vi "RobotStatus.vi"(0 "Universal Robot.lvclass in":refnum<class "Universal Robot.lvclass">, 5 "error in (no error)":errorcluster) -> (14 "Universal Robot.lvclass out":refnum<class "Universal Robot.lvclass">, 15 "Robot Status":T1, 19 "error out":errorcluster)   [LabVIEW 2019, in "Universal Robot.lvclass"]
uses:
  Universal Robot.lvclass
  RobotStatus.ctl
  RobotMode.ctl
  OperationalMode.ctl
  SafetyStatus.ctl
  Universal Robot.lvclass/Universal Robot.ctl
  Client Interfaces/Dashboard Server/Dashboard Server.lvclass
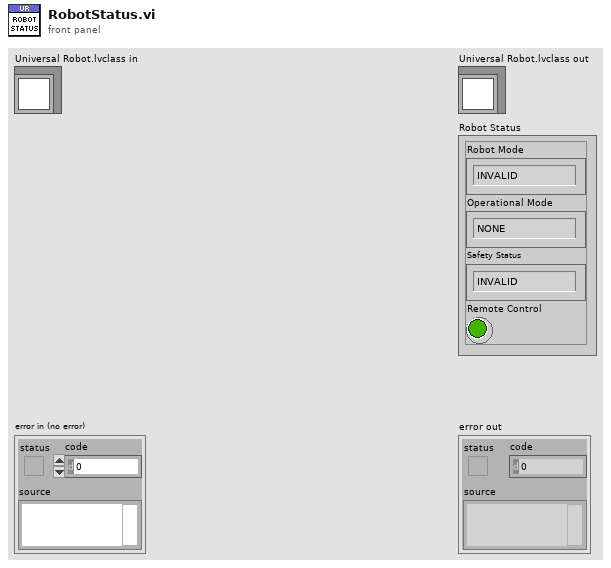
[diagram p1: front panel]
types:
  T1 = typedef "Universal Robot.lvclass/RobotStatus.ctl" = cluster{"Robot Mode":T2, "Operational Mode":T3, "Safety Status":T4, "Remote Control":bool}
  T2 = typedef "Universal Robot.lvclass/RobotMode.ctl" = enum16{"INVALID", "NO_CONTROLLER", "DISCONNECTED", "CONFIRM_SAFETY", "BOOTING", "POWER_OFF", "POWER_ON", "IDLE", "BACKDRIVE", "RUNNING"}
  T3 = typedef "Universal Robot.lvclass/OperationalMode.ctl" = enum16{"NONE", "MANUAL", "AUTOMATIC"}
  T4 = typedef "Universal Robot.lvclass/SafetyStatus.ctl" = enum16{"INVALID", "NORMAL", "REDUCED", "PROTECTIVE_STOP", "RECOVERY", "SAFEGUARD_STOP", "SYSTEM_EMERGENCY_STOP", "ROBOT_EMERGENCY_STOP", "VIOLATION", "FAULT", "AUTOMATIC_MODE_SAFEGAURD_STOP", "SYSTEM_THREE_POSITION_ENABLING_STOP"}
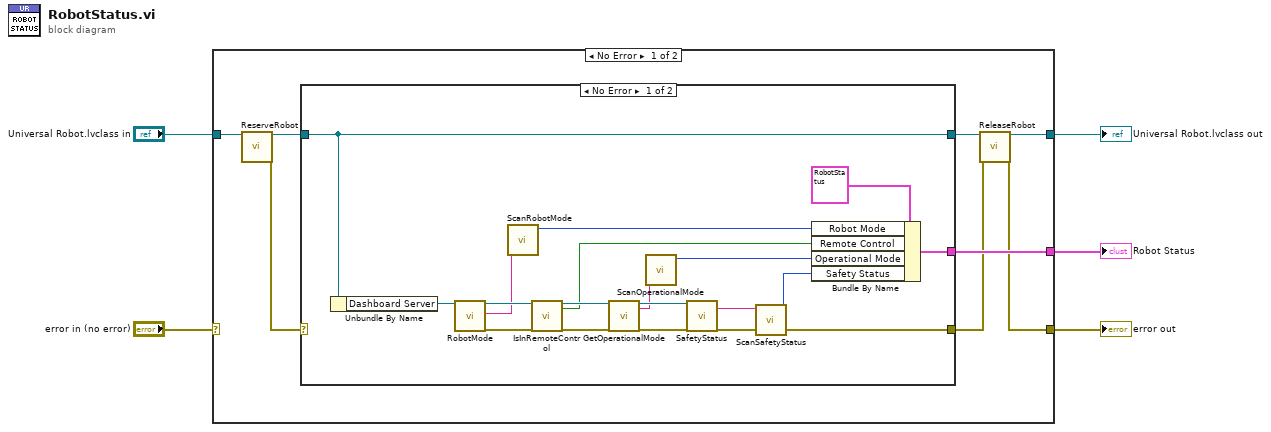
[diagram p0: block diagram]
diagram:
  n1 = case shown="No Error" "error in (no error)" {
    selector: "error in (no error)" -> [_ w35]
    tunnel: [w7 w35] -> w4
    tunnel: "Universal Robot.lvclass in" -> [w12 w34]
    tunnel: [w6 w34] -> w2
    tunnel: [w13 _] -> w1
    frame No Error {
      n2 = call "ReserveRobot.vi"("Universal Robot.lvclass in"=w12) -> ("Universal Robot.lvclass out"=w11:refnum<class "Universal Robot.lvclass">, "error out"=w10:errorcluster)  [unwired: 17 in]
      n3 = case shown="No Error" w10 {
        selector: w10 -> [_ w32]
        tunnel: [w21 _] -> w13
        tunnel: w11 -> [w14 w33]
        tunnel: [w14 w33] -> w9
        tunnel: [w15 w32] -> w8
        frame No Error {
          n4 = Unbundle By Name(w14) -> ("Dashboard Server"=w31:refnum<class "Dashboard Server.lvclass">)
          n5 = call-dynamic "RobotMode.vi"("DashboardServer in"=w31) -> ("DashboardServer out"=w30:refnum<class "Dashboard Server.lvclass">, "robotMode"=w16:string, "error out"=w27:errorcluster)  [unwired: 16 in]
          n6 = call "ScanRobotMode.vi"("robotMode in"=w16) -> ("robotMode out"=w23:T2)  [unwired: 10 in]
          n7 = call-dynamic "IsInRemoteControl.vi"("DashboardServer in"=w30, "error in (no error)"=w27) -> ("DashboardServer out"=w29:refnum<class "Dashboard Server.lvclass">, "remoteControl"=w22:bool, "error out"=w26:errorcluster)  [unwired: 15 in]
          n8 = call-dynamic "GetOperationalMode.vi"("DashboardServer in"=w29, "error in (no error)"=w26) -> ("DashboardServer out"=w28:refnum<class "Dashboard Server.lvclass">, "operationalMode"=w20:string, "error out"=w25:errorcluster)  [unwired: 15 in]
          n9 = call "ScanOperationalMode.vi"("operationalMode in"=w20) -> ("operationalMode out"=w19:T3)  [unwired: 10 in]
          n10 = call-dynamic "SafetyStatus.vi"("DashboardServer in"=w28, "error in (no error)"=w25) -> ("safetyStatus"=w18:string, "error out"=w15:errorcluster)  [unwired: 15 in, 1 out]
          n11 = call "ScanSafetyStatus.vi"("safetyStatus in"=w18) -> ("safetyStatus out"=w17:T4)  [unwired: 10 in]
          n12 = Bundle By Name(cluster=T1 {"Robot Mode"=enum."INVALID", "Operational Mode"=enum."NONE", "Safety Status"=enum."INVALID", "Remote Control"=FALSE} ("Robot Status"), "Robot Mode"=w23, "Remote Control"=w22, "Operational Mode"=w19, "Safety Status"=w17) -> (w21:T1)
        }
        frame Error {
        }
      }
      n13 = call "ReleaseRobot.vi"("Universal Robot.lvclass in"=w9, "error in (no error)"=w8) -> ("Universal Robot.lvclass out"=w6:refnum<class "Universal Robot.lvclass">, "error out"=w7:errorcluster)  [unwired: 16 in]
    }
    frame Error {
    }
  }
  "error out" <- w4
  "Universal Robot.lvclass out" <- w2
  "Robot Status" <- w1
